vi "Expand1DValues.vi"(9 "NumValues":u16[](array[numeric]), 10 "Values 1D":dbl[](array[numeric]) format="%.2f", 11 "NumFrames":i32) -> (2 "Values 2D":dbl[][](array[numeric]) format="%.2f")   [LabVIEW 2020]
panel:
  # "Takes a 1D array of values and expands it to 2D.  Number of columns will be\nthe maximum NumValues element.  Extra 9999s added as filler if needed."
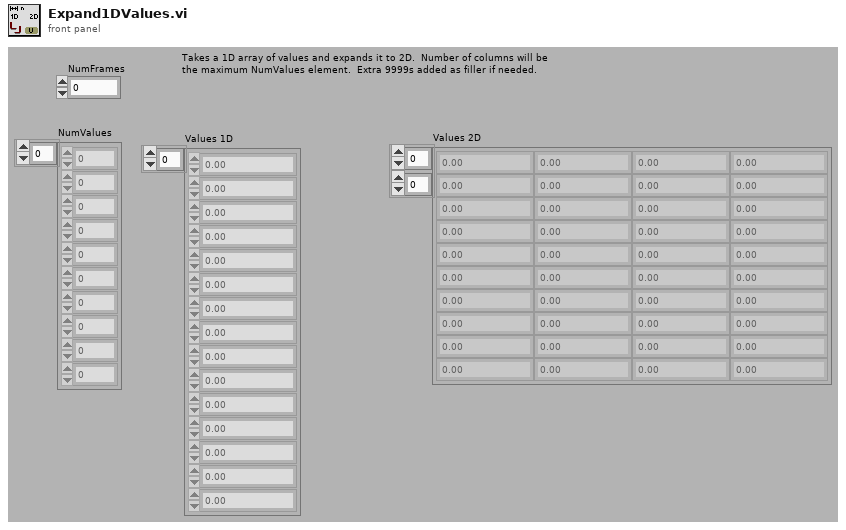
[diagram p1: front panel]
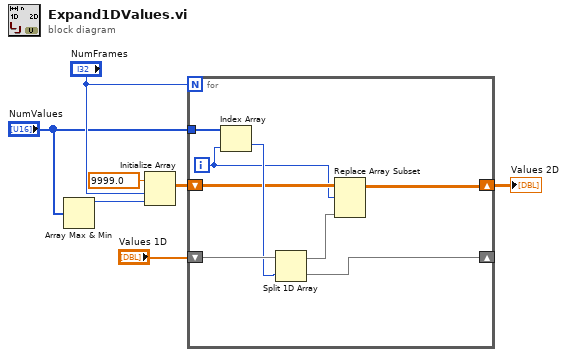
[diagram p0: block diagram]
diagram:
  n1 = Array Max & Min(array="NumValues") -> (max value=w4:u16)  [unwired: 3 out]
  n2 = Initialize Array(9999.0 ("Element Data"), "NumFrames", w4) -> (w7:dbl[][])
  n3 = for {
    N: "NumFrames" -> [_]
    shift-right: [w8] -> w1
    shift-left: w7 -> [w11]
    tunnel: "NumValues" -> [w15]
    shift-right: [w12] -> _
    shift-left: "Values 1D" -> [w14]
    i -> [w10]
    n4 = Index Array(array=w15, index=w10) -> (element=w13:u16)
    n5 = Split 1D Array(array=w14, index=w13) -> (first subarray=w9:dbl[], second subarray=w12:dbl[])
    n6 = Replace Array Subset(array=w11, new element=w9, index (row)=w10) -> (w8:dbl[][])  [unwired: 1 in]
  }
  "Values 2D" <- w1
